vi "保存二进制文件.vi"() -> ()   [LabVIEW 2010]
uses:
  <vilib>/Analysis/NI_AALBase.lvlib
panel:
  in  "stop":bool
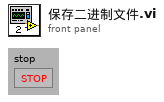
[diagram p1: front panel]
types:
  T1 = enum16{"open", "replace", "create", "open or create", "replace or create", "replace or create with confirmation"}
  T2 = enum16{"big-endian, network order", "native, host order", "little-endian"}
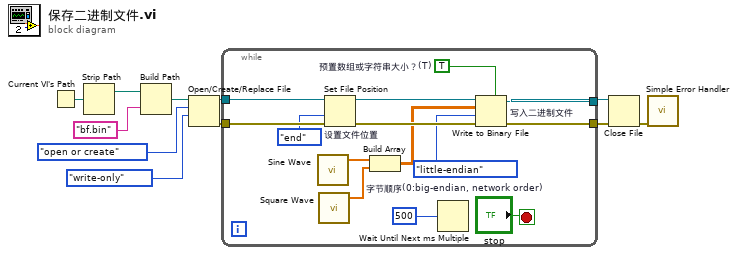
[diagram p0: block diagram]
diagram:
  n1 = Current VI's Path() -> (path=w11:path)
  n2 = Strip Path(path=w11) -> (stripped path=w6:path)  [unwired: 1 out]
  n3 = Build Path(base path=w6, name or relative path="bf.bin") -> (appended path=w5:path)
  n4 = Open/Create/Replace File(file path (use dialog)=w5, operation (0:open)=T1."open or create" ("操作(0:open)"), access (0:read/write)=enum16{"read/write", "read-only", "write-only"}."write-only" ("权限(0:read/write)")) -> (refnum out=w4:refnum<file>, error out=w3:errorcluster)  [unwired: 3 in, 1 out]
  n5 = while {
    tunnel: w3 -> [w25]
    tunnel: [w23] -> w9
    tunnel: [w22] -> w8
    tunnel: w4 -> [w16]
    stop <- "stop" stop-if-true
    w12 = T2."little-endian"  # 字节顺序(0:big-endian, network order)
    w17 = TRUE  # 预置数组或字符串大小？(T)
    n6 = call <vilib>:"Sine Wave.vi"() -> ("sine wave"=w15:dbl[])  [unwired: 5 in, 2 out]
    n7 = call <vilib>:"Square Wave.vi"() -> ("square wave"=w14:dbl[])  [unwired: 6 in, 2 out]
    n8 = Set File Position "设置文件位置"(refnum=w16, from (0:start)=enum16{"start", "end", "current"}."end" ("pos mode (0:2)"), error in=w25) -> (refnum out=w19:refnum<file>, error out=w18:errorcluster)  [unwired: 1 in]
    n9 = Build Array(w15, w14) -> (w13:dbl[][])
    n10 = Wait Until Next ms Multiple(millisecond multiple=u32 500) -> ()  [unwired: 1 out]
    n11 = Write to Binary File "写入二进制文件"(file (use dialog)=w19, data=w13, error in=w18, 5:w17, 9:w12) -> (refnum out=w23:refnum<file>, error out=w22:errorcluster)  [unwired: 1 in, 1 out]
  }
  n12 = Close File(refnum=w9, error in=w8) -> (error out=w7:errorcluster)  [unwired: 1 out]
  n13 = call <vilib>:"Simple Error Handler.vi"("error in (no error)"=w7) -> ()  [unwired: 4 in, 5 out]
